vi "Calculate Control Position.vi"(0 "size array":u32[][](array[numeric])) -> (2 "position array":u32[](array[numeric]), 3 "sum value":i16)   [LabVIEW 2018, in "NISAST VI Scripting.lvlib" / "VI.lvlib" / "Front Panel.lvlib"]
uses:
  Front Panel.lvlib
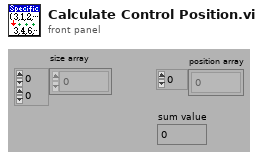
[diagram p1: front panel]
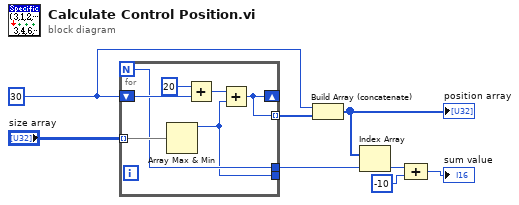
[diagram p0: block diagram]
diagram:
  w5 = u32 30
  n1 = for {
    N -> [w10]
    tunnel: "size array" -> [w15] mode=indexing
    shift-right: [w11] -> _
    shift-left: w5 -> [w14]
    tunnel: [w11] -> w7 mode=indexing
    tunnel: [w10] -> w4
    tunnel: [w9] -> _
    n2 = Array Max & Min(array=w15) -> (max value=w9:u32)  [unwired: 3 out]
    n3 = Add(x=u32 20, y=w14) -> (x+y=w12:u32)
    n4 = Add(x=w12, y=w9) -> (x+y=w11:u32)
  }
  n5 = Build Array (concatenate)(w5, w7) -> (w6:u32[])
  "position array" <- w6
  n6 = Index Array(array=w6, index=w4) -> (element=w1:u32)
  n7 = Compound Arithmetic op=ADD(w1, -10 ("Input")) -> (→"sum value":u32)
